vi "Move to Cartisean.vi"(4 "Tolerance":dbl=1.0, 6 "Step":dbl=25.0, 7 "Side":T1=enum."right", 8 "error in":errorcluster, 10 "to Goal":bool, 11 "Goal":T2={"X"=600.0, "Y"=200.0, "Z"=0.0, "Roll"=0.0, "Pitch"=0.0, "Yaw"=180.0}) -> (0 "error out":errorcluster, 2 "Found":bool, 3 "At Goal":bool=TRUE)   [LabVIEW 2013]
uses:
  BaxterVIs/Command_Joint_Angles.vi
  BaxterVIs/Read_Joint_States_A.vi
  Cartesian/Goal.ctl
  ROS/Code/SubVIs/BaxterSide.ctl
panel:
  out "Close":bool
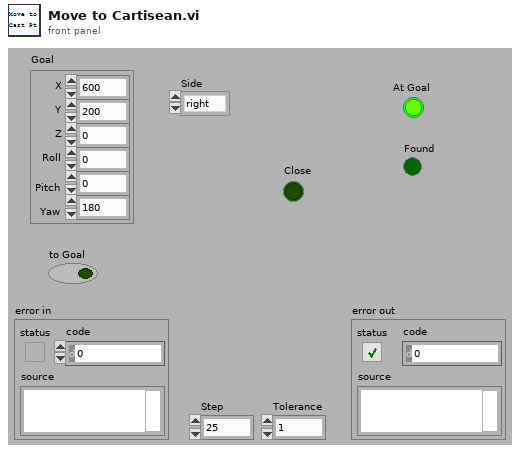
[diagram p1: front panel]
types:
  T1 = typedef "BaxterSide.ctl" = enum16{"left", "right"}
  T2 = typedef "Goal.ctl" = cluster{"X":dbl, "Y":dbl, "Z":dbl, "Roll":dbl, "Pitch":dbl, "Yaw":dbl}
  T3 = typedef "NI_Matrix.lvlib/RealMatrix.ctl" = dbl[][]
  T4 = typedef "BaxterArmsSmall.ctl" = cluster{"Elbow 0":dbl, "Elbow 1":dbl, "Shoulder 0":dbl, "Shoulder 1":dbl, "Wrist 0":dbl, "Wrist 1":dbl, "Wrist 2":dbl}
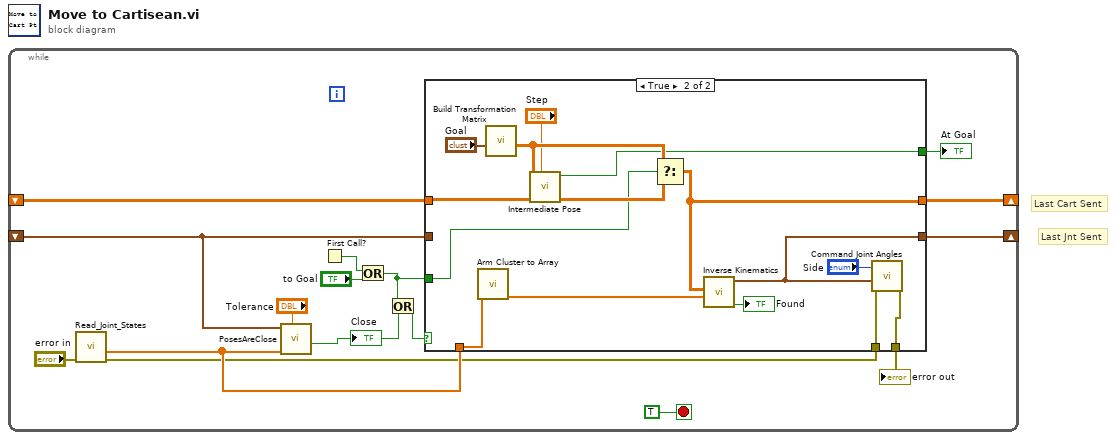
[diagram p0: block diagram]
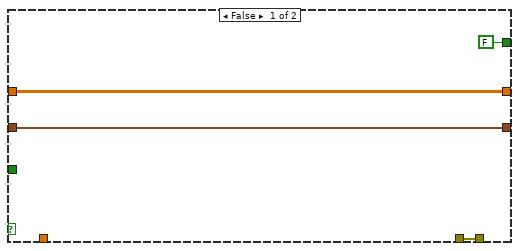
[diagram p2: hidden frame]
diagram:
  # "Last Jnt Sent"
  # "Last Cart Sent"
  n1 = while {
    shift-right: [w15] -> _
    shift-left: _ -> [w11]
    shift-right: [w10] -> _
    shift-left: _ -> [w9]
    stop <- TRUE stop-if-true
    n2 = call-poly "Read_Joint_States.vi"("error in"="error in") -> ("error out"=w12:errorcluster, "right Positions"=w13:dbl[])  [unwired: 4 in, 2 out]
    n3 = call "PosesAreClose.vi"("Tolerance"="Tolerance", "Position 2"=w13, "Position"=w11) -> ("Close"=w6:bool)  [unwired: 8 in]
    "Close" <- w6
    n4 = First Call?() -> (First Call?: T/F=w2:bool)
    n5 = Or(x=w2, y="to Goal") -> (x .or. y?=w3:bool)
    n6 = Or(x=w3, y=w6) -> (x .or. y?=w5:bool)
    n7 = case shown="True" w5 {
      tunnel: [w19 w30] -> w15
      tunnel: w12 -> [w20 w35]
      tunnel: [w20 w34] -> w16
      tunnel: w11 -> [w19 _]
      tunnel: w13 -> [_ w32]
      tunnel: [w18 w25] -> w10
      tunnel: w9 -> [w18 w28]
      tunnel: w3 -> [_ w22]
      tunnel: [FALSE ("At Goal") w21] -> w1
      frame False {
      }
      frame True {
        n8 = call "Arm Cluster to Array.vi"("Current"=w32) -> ("Joints"=w31:dbl[])  [unwired: 10 in]
        n9 = call "Build Transformation Matrix.vi"("Goal"="Goal") -> ("T"=w27:T3)  [unwired: 10 in]
        n10 = call "Intermediate Pose.vi"("Step"="Step", "Last Pose"=w28, "Goal"=w27) -> ("Pose"=w26:T3, "At Goal"=w21:bool)  [unwired: 7 in]
        n11 = Select(t=w27, s=w22, f=w26) -> (s? t:f=w25:T3)
        n12 = call "Inverse Kinematics.vi"("Start"=w31, "Goal-matrix"=w25) -> ("Found"=→"Found":bool, "Arm Angles"=w30:T4)  [unwired: 6 in, 2 out]
        n13 = call-poly "Command Joint Angles.vi"("error in"=w35, "Arm Angles (degrees)"=w30, "Side"="Side") -> ("error out"=w34:errorcluster)  [unwired: 6 in]
      }
    }
    "error out" <- w16
    "At Goal" <- w1
  }
